vi "Instrument.OxfordVRM.FloatApprox.vi"(4 "y":dbl, 5 "x":dbl) -> (1 "x ~ y?":bool)   [LabVIEW 2019, in "Instrument.OxfordVRM.lvclass"]
doc: "Use to compare floating point numbers. This will check if two numbers are the same to 6 decimal places. Edit block diagram to change tolerance."
uses:
  Instrument.OxfordVRM.lvclass
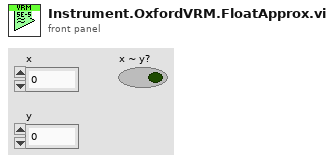
[diagram p1: front panel]
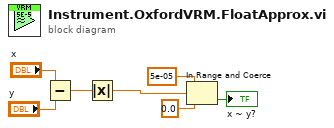
[diagram p0: block diagram]
diagram:
  n1 = Subtract(x="x", y="y") -> (x-y=w4:dbl)
  n2 = Absolute Value(x=w4) -> (abs(x)=w1:dbl)
  n3 = In Range and Coerce(upper limit=5e-05, x=w1, lower limit=0.0 ("upper limit")) -> (In Range?=→"x ~ y?":bool)  [unwired: 1 out]
